vi "Fatima_test.vi"() -> ()   [LabVIEW 2020]
uses:
  LightField Automation.lvclass
panel:
  in  "Boolean":bool
  out "ROI 1, Frame 1, Row 1":dbl[](graph)
  out "ROI 1, Frame 1":dbl[][](graph)
  out "Data":T1(array[cluster])
  in  "stop":bool
  in  "Exposure Time (s)":dbl
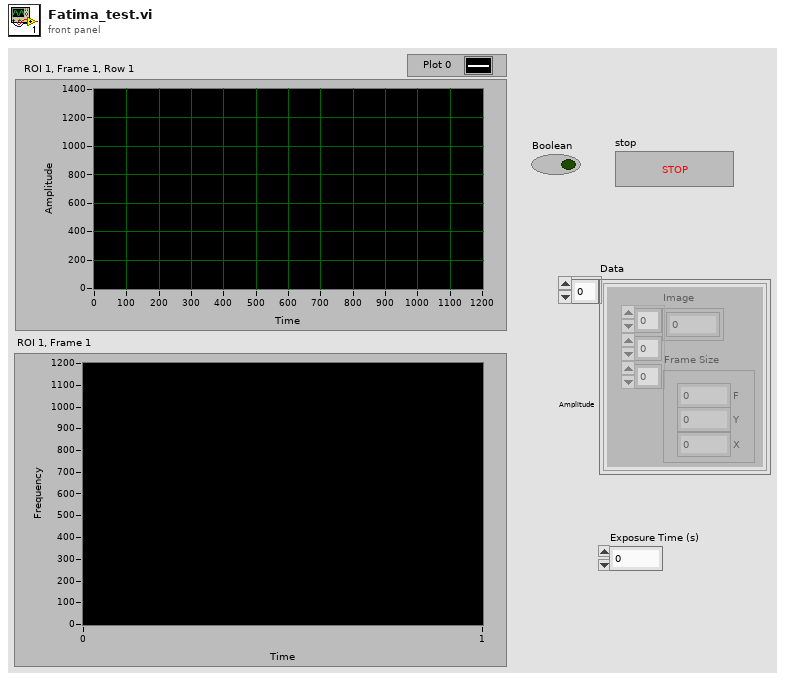
[diagram p1: front panel]
types:
  T1 = cluster{"Image":dbl[][][], "Frame Size":cluster{"F":i32, "Y":i32, "X":i32}}[]
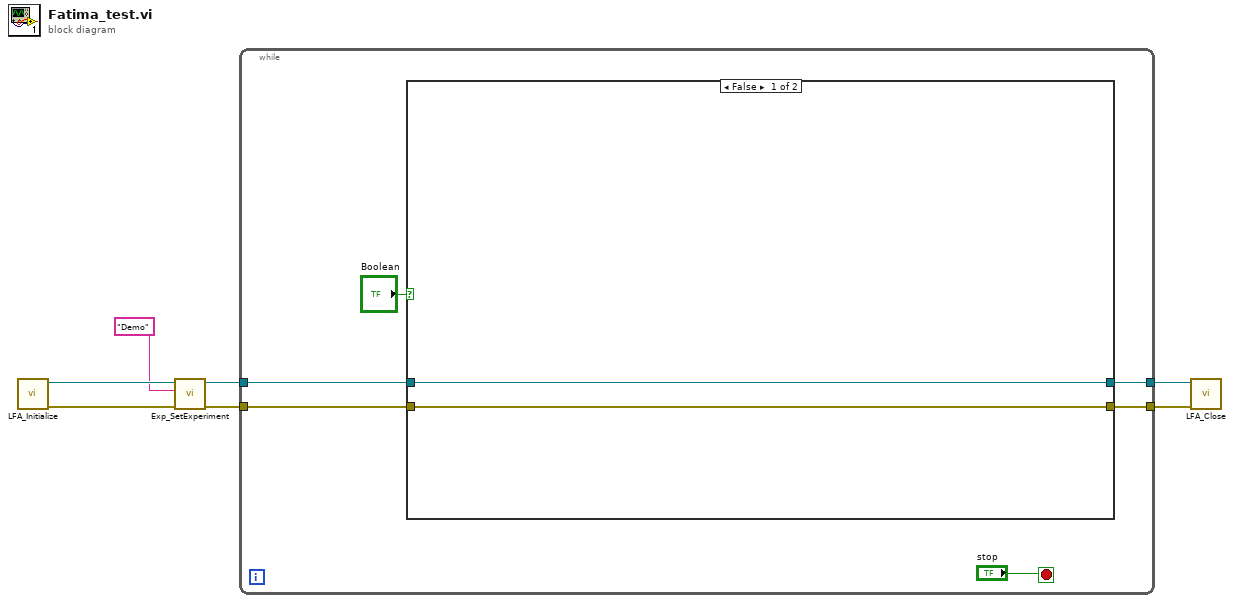
[diagram p0: block diagram]
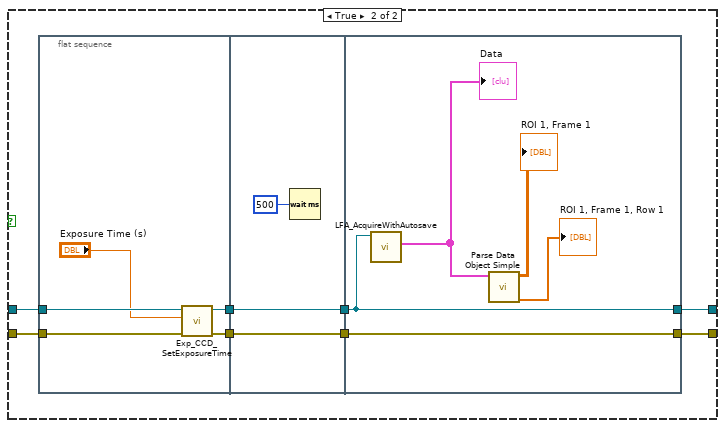
[diagram p2: hidden frame]
diagram:
  n1 = call "LFA_Initialize.vi"() -> ("error out"=w7:errorcluster, "LightField Automation out"=w6:refnum<class "LightField Automation.lvclass">)  [unwired: 10 in]
  n2 = call "Exp_SetExperiment.vi"("error in (no error)"=w7, "ExperimentName"="Demo", "LightField Automation in"=w6) -> ("error out"=w4:errorcluster, "LightField Automation out"=w3:refnum<class "LightField Automation.lvclass">)  [unwired: 7 in]
  n3 = while {
    tunnel: w4 -> [w13]
    tunnel: w3 -> [w12]
    tunnel: [w10] -> w2
    tunnel: [w9] -> w1
    stop <- "stop" stop-if-true
    n4 = case shown="False" "Boolean" {
      tunnel: w13 -> [w14 w19]
      tunnel: w12 -> [w15 w18]
      tunnel: [w14 w17] -> w10
      tunnel: [w15 w16] -> w9
      frame False {
      }
      frame True {
        n5 = flat-sequence {
          tunnel: w19 -> [w28]
          tunnel: w18 -> [w27]
          tunnel: [w25] -> w23
          tunnel: [w24] -> w22
          tunnel: w23 -> [w31]
          tunnel: [w31] -> w21
          tunnel: w22 -> [w30]
          tunnel: [w30] -> w20
          tunnel: [w32] -> w16
          tunnel: [w36] -> w17
          tunnel: w21 -> [w36]
          tunnel: w20 -> [w32]
          frame #0 {
            n6 = call "Exp_CCD_SetExposureTime.vi"("error in (no error)"=w28, "Exposure Time (s)"="Exposure Time (s)", "LightField Automation in"=w27) -> ("error out"=w25:errorcluster, "LightField Automation out"=w24:refnum<class "LightField Automation.lvclass">)  [unwired: 7 in]
          }
          frame #1 {
            n7 = Wait (ms)(milliseconds to wait=u32 500 ("millisecond timer value")) -> ()  [unwired: 1 out]
          }
          frame #2 {
            n8 = call "LFA_AcquireWithAutosave.vi"("LightField Automation in"=w32) -> ("Data"=w35:T1)  [unwired: 8 in, 2 out]
            "Data" <- w35
            n9 = call "Parse Data Object Simple.vi"("Data"=w35) -> ("ROI 1, Frame 1, Row 1"=→"ROI 1, Frame 1, Row 1":dbl[], "ROI 1, Frame 1"=→"ROI 1, Frame 1":dbl[][])  [unwired: 9 in]
          }
        }
      }
    }
  }
  n10 = call "LFA_Close.vi"("error in (no error)"=w2, "LightField Automation in"=w1) -> ()  [unwired: 8 in, 2 out]
